vi "run_data_splitter.vi"(0 "Run Data":T2) -> (3 "Run Settings":T1={"Operator"="", "Sample (or CRM) ID"="", "Sample Temp"=0.0, "Salinity"=0.0, "Sample Units"=FALSE, "Sample Size"=0.0, "Operation Mode"=TRUE})   [LabVIEW 2010]
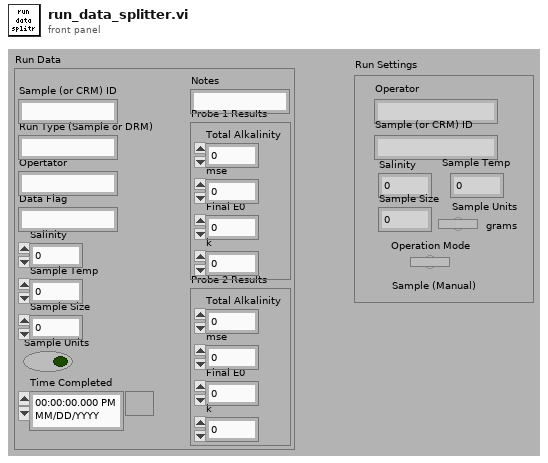
[diagram p1: front panel]
types:
  T1 = cluster{"Operator":string, "Sample (or CRM) ID":string, "Sample Temp":dbl, "Salinity":dbl, "Sample Units":bool, "Sample Size":dbl, "Operation Mode":bool}
  T2 = cluster{"Sample (or CRM) ID":string, "Run Type (Sample or DRM)":string, "Opertator":string, "Data Flag":string, "Salinity":dbl, "Sample Temp":dbl, "Sample Size":dbl, "Sample Units":bool, "Time Completed":timestamp, "Notes":string, "Probe 1 Results":cluster{"Total Alkalinity":dbl, "mse":dbl, "Final E0":dbl, "k":dbl}, "Probe 2 Results":cluster{"Total Alkalinity":dbl, "mse":dbl, "Final E0":dbl, "k":dbl}}
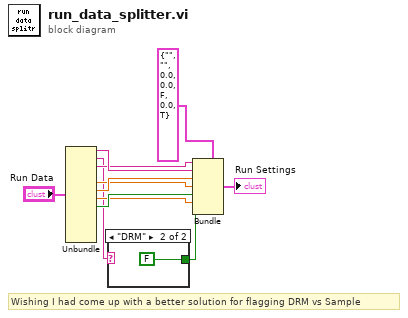
[diagram p0: block diagram]
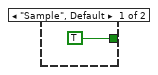
[diagram p2: hidden frame]
diagram:
  # "Wishing I had come up with a better solution for flagging DRM vs Sample"
  n1 = Unbundle("Run Data") -> ("Sample (or CRM) ID"=w8:string, "Run Type (Sample or DRM)"=w2:string, "Opertator"=w7:string, "Salinity"=w5:dbl, "Sample Temp"=w6:dbl, "Sample Size"=w3:dbl, "Sample Units"=w4:bool)  [unwired: 5 out]
  n2 = case shown="\"DRM\"" w2 {
    tunnel: [TRUE FALSE] -> w1
    frame "Sample", Default {
    }
    frame "DRM" {
    }
  }
  n3 = Bundle(cluster=T1 {"Operator"="", "Sample (or CRM) ID"="", "Sample Temp"=0.0, "Salinity"=0.0, "Sample Units"=FALSE, "Sample Size"=0.0, "Operation Mode"=TRUE} ("Run Settings"), "Operator"=w7, "Sample (or CRM) ID"=w8, "Sample Temp"=w6, "Salinity"=w5, "Sample Units"=w4, "Sample Size"=w3, "Operation Mode"=w1) -> (→"Run Settings":T1)
